vi "MPM_Get_Range_Each_for_Channel.vi"(8 "error in (no error)":errorcluster, 9 "channelNumber":i32, 10 "moduleNumber":i32, 11 ".NET Reference in":refnum<k24>) -> (0 "error out":errorcluster, 2 "range out":i32, 3 "Reference out":refnum<k24>)   [LabVIEW 2017]
doc: "Get Range for each ch"
uses:
  C:/Users/Ssantec_Test/Documents/Instrument_DLL_Sample_Labview_20220902_Ver1.2.2/DLL/x86/InstrumentDLL.dll
  DLL/x86/InstrumentDLL.dll
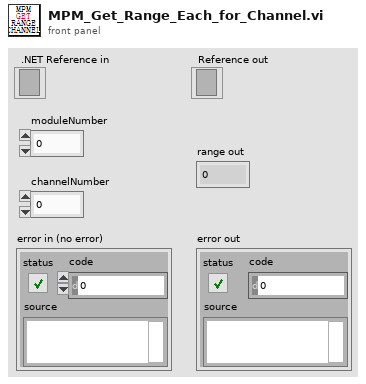
[diagram p1: front panel]
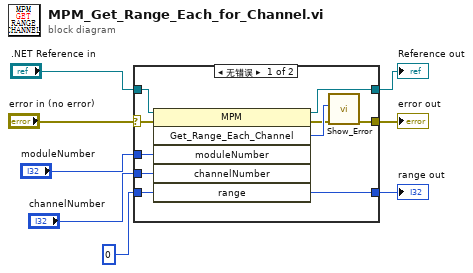
[diagram p0: block diagram]
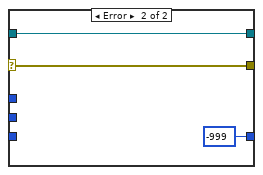
[diagram p2: hidden frame]
diagram:
  n1 = case shown="无错误" "error in (no error)" {
    selector: "error in (no error)" -> [w9 w21]
    tunnel: [w18 -999 ("range")] -> w8
    tunnel: "channelNumber" -> [w17 _]
    tunnel: "moduleNumber" -> [w16 _]
    tunnel: ".NET Reference in" -> [w15 w20]
    tunnel: [w14 w20] -> w4
    tunnel: 0 ("range") -> [w13 _]
    tunnel: [w10 w21] -> w2
    frame No Error {
      n2 = invoke on="调用节点" class="MPM" method="Get_Range_Each_Channel"(reference=w15, error in=w9, "moduleNumber"=w16, "channelNumber"=w17, "range"=w13) -> (reference out=w14:refnum<k24>, error out=w11:errorcluster, "Get_Range_Each_Channel"=w12:i32, "range"=w18:i32)  [unwired: 1 in, 2 out]
      n3 = call "Show_Error.vi"("error in (no error)"=w11, "Error"=w12) -> ("error out"=w10:errorcluster)  [unwired: 9 in]
    }
    frame Error {
    }
  }
  "range out" <- w8
  "Reference out" <- w4
  "error out" <- w2
